vi "Template Get Templates from List.vi"(8 "error in (no error)":errorcluster, 10 "sxTemplateId List(\"\")":string, 11 "Connection Refnum":T2) -> (0 "error out":errorcluster, 1 "new Templates CSV":string, 2 "Templates":T1[](array[typedef]), 3 "Connection Refnum":T2)   [LabVIEW 2011]
uses:
  Summitek EXT/ODBC/SQL Controls/Connection Refnum.ctl
  Template Record.ctl
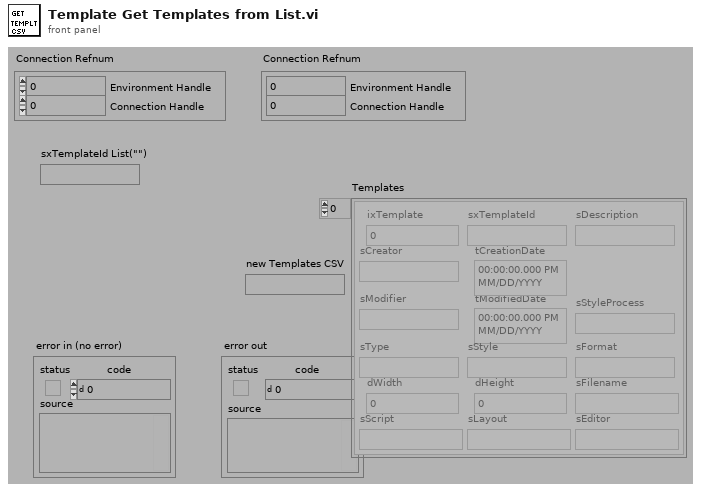
[diagram p1: front panel]
types:
  T1 = typedef "Template Record.ctl" = cluster{"ixTemplate":i32, "sxTemplateId":string, "sDescription":string, "sCreator":string, "tCreationDate":timestamp, "sModifier":string, "tModifiedDate":timestamp, "sType":string, "sStyle":string, "sFormat":string, "dWidth":dbl, "dHeight":dbl, "sFilename":string, "sScript":string, "sLayout":string, "sEditor":string, "sStyleProcess":string}
  T2 = typedef "Connection Refnum.ctl" = cluster{"Environment Handle":i32, "Connection Handle":i32}
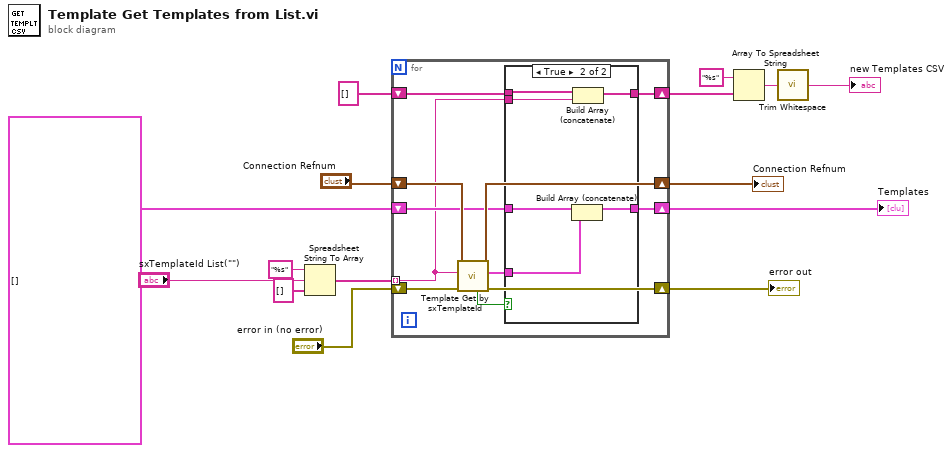
[diagram p0: block diagram]
diagram:
  n1 = Spreadsheet String To Array(format string="%s", spreadsheet string="sxTemplateId List(\"\")", array type (2D Dbl)=string[] []) -> (array=w3:string[])  [unwired: 1 out]
  n2 = for {
    shift-right: [w25] -> w11
    shift-left: "error in (no error)" -> [w26]
    tunnel: w3 -> [w16] mode=indexing
    shift-right: [w23] -> w12
    shift-left: "Connection Refnum" -> [w24]
    shift-right: [w19] -> w10
    shift-left: T1[] [] -> [w21]
    shift-right: [w17] -> w6
    shift-left: string[] [] -> [w18]
    n3 = call "Template Get by sxTemplateId.vi"("error in (no error)"=w26, "sxTemplateId (\"\")"=w16, "Connection Refnum"=w24) -> ("error out"=w25:errorcluster, "Template Record"=w20:T1, "Connection Refnum"=w23:T2, "Data Present"=w22:bool)  [unwired: 5 out]
    n4 = case shown="True" w22 {
      tunnel: w21 -> [w28 w34]
      tunnel: w20 -> [_ w33]
      tunnel: [w28 w32] -> w19
      tunnel: w18 -> [w27 w31]
      tunnel: [w27 w30] -> w17
      tunnel: w16 -> [_ w29]
      frame False {
      }
      frame True {
        n5 = Build Array (concatenate)(w34, w33) -> (w32:T1[])
        n6 = Build Array (concatenate)(w31, w29) -> (w30:string[])
      }
    }
  }
  "error out" <- w11
  "Connection Refnum" <- w12
  "Templates" <- w10
  n7 = Array To Spreadsheet String(array=w6, 3:"%s" ("format string")) -> (spreadsheet string=w7:string)  [unwired: 1 out]
  n8 = call <vilib>:"Trim Whitespace.vi"("string"=w7) -> ("trimmed string"=→"new Templates CSV":string)  [unwired: 1 in]
